vi "receive_03proc.vi"() -> ()   [LabVIEW 2015]
uses:
  <instrlib>/niUSRP/niUSRP Fetch Rx Data (CDB Cluster).vi
  <vilib>/Waveform/WDTOps.llb/WDT Get Waveform Subset DBL.vi
panel:
  in  "duration":dbl=180.0 format="%#_13g"
  in  "start":i64=570 format="%.0g"
  out "error out 2":errorcluster
  out "duration":dbl format="%0.2f"
  out "start samples":dbl format="%0.2f"
  out "Portion Signal":waveform(dbl)(graph)
  out "Filename Out":path
  out "Saving Data":bool
  out "Triggered Signal":dynamicdata(graph)
  out "Data Available":bool
  in  "active antenna":string="RX2"
  in  "Channels":string(combo)="0"
  out "Magnitude":cluster{"t0":dbl, "dt":dbl, "Y":dbl[]}(graph)
  in  "Stop":bool
  out "coerced gain":dbl format="%#_6f"
  out "coerced carrier frequency":dbl=100000.0 format="%#_6p"
  out "coerced IQ rate":dbl=100000.0 format="%#_6p"
  in  "gain":dbl format="%#_6f"
  in  "carrier frequency":dbl=920000000.0 format="%#_6p"
  in  "IQ rate":dbl=2000000.0 format="%#_6p"
  in  "number of samples":i64=2000000
  in  "timeout":dbl=10.0
  out "error out":errorcluster
  in  "device names":refnum<k15>="192.168.10.14"
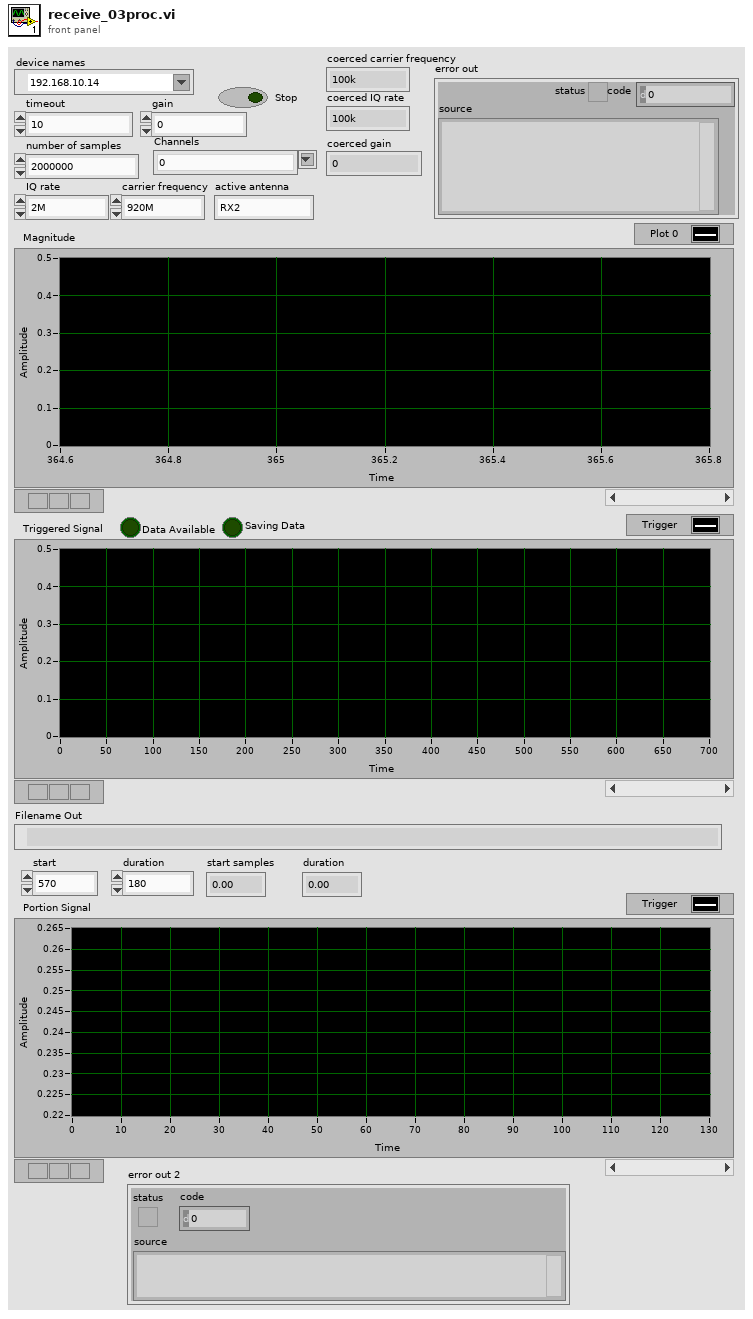
[diagram p1: front panel]
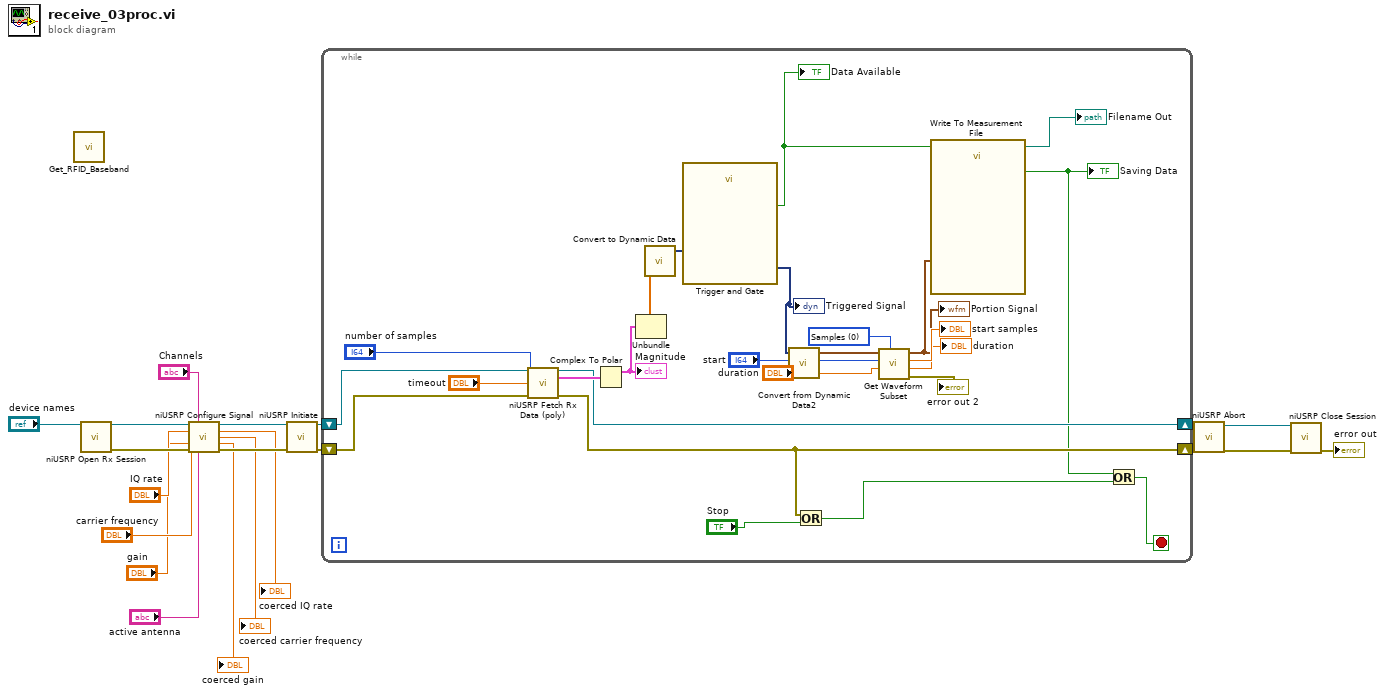
[diagram p0: block diagram]
diagram:
  n1 = call "Get_RFID_Baseband.vi"() -> ()  [unwired: 14 in, 2 out]
  n2 = call <instrlib>:"niUSRP Open Rx Session.vi"("device names"="device names") -> ("session handle out"=w19:refnum<k15>, "error out"=w18:errorcluster)  [unwired: 13 in]
  n3 = call <instrlib>:"niUSRP Configure Signal.vi"("session handle"=w19, "channel list"="Channels", "IQ rate"="IQ rate", "carrier frequency"="carrier frequency", "gain"="gain", "error in (no error)"=w18, "active antenna"="active antenna") -> ("session handle out"=w17:refnum<k15>, "coerced IQ rate"=→"coerced IQ rate":dbl, "coerced carrier frequency"=→"coerced carrier frequency":dbl, "coerced gain"=→"coerced gain":dbl, "error out"=w16:errorcluster)  [unwired: 4 in]
  n4 = call <instrlib>:"niUSRP Initiate.vi"("session handle"=w17, "error in (no error)"=w16) -> ("session handle out"=w15:refnum<k15>, "error out"=w14:errorcluster)  [unwired: 12 in]
  n5 = while {
    shift-right: [w41] -> w13
    shift-left: w15 -> [w40]
    shift-right: [w38] -> w12
    shift-left: w14 -> [w39]
    stop <- w32 stop-if-true
    w27 = u16 0 items=["Samples", "Relative Time"] ("start/duration format")
    n6 = call-poly <instrlib>:"niUSRP Fetch Rx Data (poly).vi"("session handle"=w40, "number of samples"="number of samples", "timeout"="timeout", "error in (no error)"=w39) -> ("session handle out"=w41:refnum<k15>, "data"=w42:cluster{"t0":dbl, "dt":dbl, "Y":cdb[]}, "error out"=w38:errorcluster)  [unwired: 8 in, 1 out]
    n7 = Complex To Polar(r * e^(i*theta)=w42) -> (r=w37:cluster{"t0":dbl, "dt":dbl, "Y":dbl[]})  [unwired: 1 out]
    "Magnitude" <- w37
    n8 = Unbundle(w37) -> ("Y"=w30:dbl[])  [unwired: 2 out]
    n9 = call "Convert to Dynamic Data"("Array"=w30) -> ("Dynamic Data Type"=w36:dynamicdata)  [unwired: 3 in]
    n10 = call "Trigger and Gate"("Signals"=w36) -> ("Triggered Signals"=w24:dynamicdata, "Data Available"=w35:bool)  [unwired: 7 in, 2 out]
    "Data Available" <- w35
    "Triggered Signal" <- w24
    n11 = call "Convert from Dynamic Data2"("Dynamic Data Type"=w24) -> ("Waveform"=w23:waveform(dbl))  [unwired: 3 in]
    n12 = Or(x=w38, y="Stop") -> (x .or. y?=w33:bool)
    n13 = call-poly <vilib>:"Get Waveform Subset.vi"("start/duration format"=w27, "duration"="duration", "start samples/time"="start", "waveform in"=w23) -> ("error out"=→"error out 2":errorcluster, "actual duration"=→"duration":dbl, "actual start samples/time"=→"start samples":dbl, "waveform out"=w21:waveform(dbl))  [unwired: 2 in]
    "Portion Signal" <- w21
    n14 = call "Write To Measurement File"("Signals"=w21, "Enable"=w35) -> ("Filename Out"=→"Filename Out":path, "Saving Data"=w31:bool)  [unwired: 15 in, 1 out]
    "Saving Data" <- w31
    n15 = Or(x=w31, y=w33) -> (x .or. y?=w32:bool)
  }
  n16 = call <instrlib>:"niUSRP Abort.vi"("session handle"=w13, "error in (no error)"=w12) -> ("session handle out"=w11:refnum<k15>, "error out"=w10:errorcluster)  [unwired: 12 in]
  n17 = call <instrlib>:"niUSRP Close Session.vi"("session handle"=w11, "error in (no error)"=w10) -> ("error out"=→"error out":errorcluster)  [unwired: 13 in]
